vi "Refresh Dependent Modules.vi"(8 "error in (no error)":errorcluster, 11 "Routing and Faulting Ref in":T1 format="%.0x") -> (0 "error out":errorcluster, 3 "Routing and Faulting Ref out":T1 format="%.0x")   [LabVIEW 2017, in "Routing and Faulting Scripting.lvlib"]
uses:
  <vilib>/NI Veristand/Custom Device API/Custom Device Item Ref.ctl
  Routing and Faulting Scripting.lvlib
  Shared/Routing and Faulting Hardware API/Routing and Faulting Hardware API.lvlib
  System Explorer/Routing and Faulting System Explorer.lvlib
  <vilib>/NI Veristand/Custom Device API/Custom Device API.lvlib
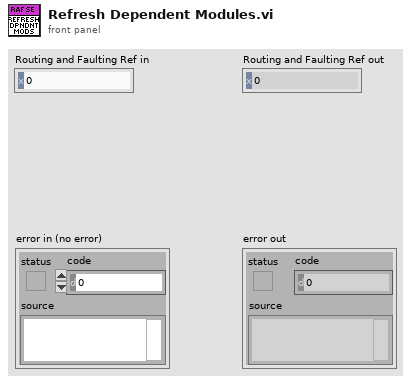
[diagram p1: front panel]
types:
  T1 = typedef "Custom Device API.lvlib/Custom Device Item Ref.ctl" = u64
  T2 = cluster{"Expected Path":string, "Module Ref":T1}[]
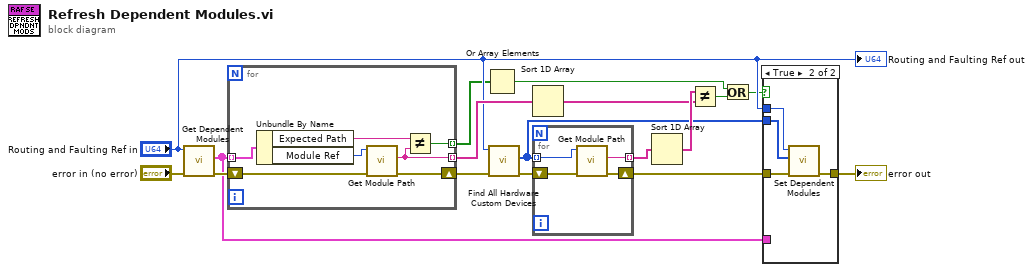
[diagram p0: block diagram]
diagram:
  n1 = call "Get Dependent Modules.vi"("error in (no error)"="error in (no error)", "Routing and Faulting Ref in"="Routing and Faulting Ref in") -> ("error out"=w15:errorcluster, "Dependent Modules"=w8:T2)  [unwired: 7 in, 1 out]
  n2 = for {
    tunnel: w8 -> [w24] mode=indexing
    shift-right: [w21] -> w12
    shift-left: w15 -> [w22]
    tunnel: [w19] -> w14 mode=indexing
    tunnel: [w18] -> w2 mode=indexing
    n3 = Unbundle By Name(w24) -> ("Expected Path"=w20:string, "Module Ref"=w23:T1)
    n4 = call "Get Module Path.vi"("error in (no error)"=w22, "Hardware Ref in"=w23) -> ("error out"=w21:errorcluster, "Resource"=w19:string)  [unwired: 6 in, 2 out]
    n5 = Not Equal?(x=w20, y=w19) -> (x != y?=w18:bool)
  }
  n6 = Or Array Elements(Boolean array=w2) -> (logical OR=w1:bool)
  n7 = call "Find All Hardware Custom Devices.vi"("error in (no error)"=w12, "Routing and Faulting Ref in"="Routing and Faulting Ref in") -> ("error out"=w16:errorcluster, "Hardware Refs"=w6:T1[])  [unwired: 7 in, 1 out]
  n8 = Sort 1D Array(array=w14) -> (sorted array=w10:string[])
  n9 = for {
    tunnel: w6 -> [w28] mode=indexing
    tunnel: [w26] -> w13 mode=indexing
    shift-right: [w25] -> w9
    shift-left: w16 -> [w27]
    n10 = call "Get Module Path.vi"("error in (no error)"=w27, "Hardware Ref in"=w28) -> ("error out"=w25:errorcluster, "Resource"=w26:string)  [unwired: 6 in, 2 out]
  }
  n11 = Sort 1D Array(array=w13) -> (sorted array=w11:string[])
  n12 = Not Equal?(x=w11, y=w10) -> (x != y?=w4:bool)
  n13 = Or(x=w1, y=w4) -> (x .or. y?=w3:bool)
  n14 = case shown="True" w3 {
    tunnel: w9 -> [w29 w32]
    tunnel: w8 -> [_ _]
    tunnel: "Routing and Faulting Ref in" -> [_ w31]
    tunnel: [w29 w33] -> w5
    tunnel: w6 -> [_ w30]
    frame False {
    }
    frame True {
      n15 = call "Set Dependent Modules.vi"("error in (no error)"=w32, "Dependent Module Refs"=w30, "Routing and Faulting Ref in"=w31) -> ("error out"=w33:errorcluster)  [unwired: 7 in, 1 out]
    }
  }
  "error out" <- w5
  "Routing and Faulting Ref out" <- "Routing and Faulting Ref in"
